vi "Update Named Tag.vi"(7 "Index":i32, 8 "error in (no error)":errorcluster, 9 "Variant":variant, 10 "Tag Name":string, 11 "Raw Message in":refnum<class "Raw Message.lvclass">) -> (0 "error out":errorcluster, 2 "Key not found?":bool, 3 "Raw Message out":refnum<class "Raw Message.lvclass">)   [LabVIEW 2020]
uses:
  Raw Message.lvclass/Raw Message.ctl
  Tag/Basic Type.lvclass
  Raw Message.lvclass
  E:/Labview/LV 2020/Libs/LV Protobuf Raw/Source/Tag/Basic Type.lvclass
  E:/Labview/LV 2020/Libs/LV Protobuf Raw/Source/Proto Value/Proto Type.lvclass
  E:/Labview/LV 2020/Libs/LV Protobuf Raw/Source/Type Serializer/Type Serializer.lvclass
  E:/Labview/LV 2020/Libs/LV Protobuf Raw/Source/String Representable/String Representable.lvclass
  E:/Labview/LV 2020/Libs/LV Protobuf Raw/Source/Wire Type Group/Wire Type Group.lvclass
  E:/Labview/LV 2020/Libs/LV Protobuf Raw/Source/LEN Encoder/LEN.lvclass
  E:/Labview/LV 2020/Libs/LV Protobuf Raw/Source/Message/Raw Message.lvclass
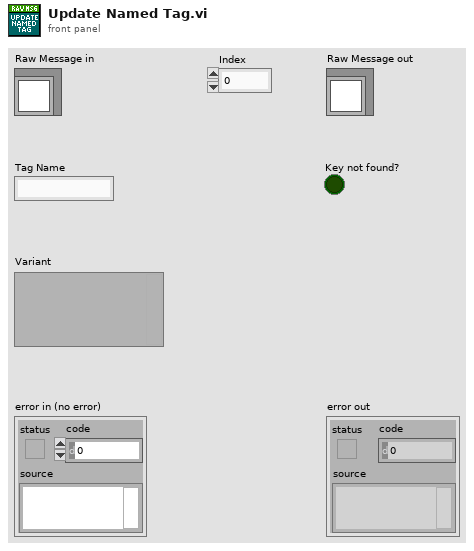
[diagram p1: front panel]
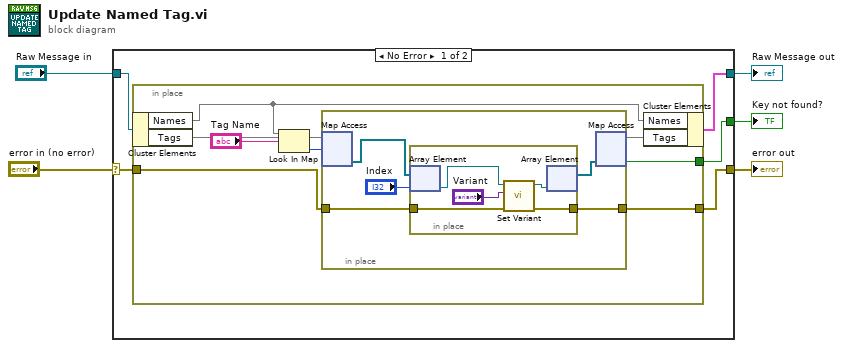
[diagram p0: block diagram]
diagram:
  n1 = case shown="No Error" "error in (no error)" {
    selector: "error in (no error)" -> [w8 w30]
    tunnel: [w7 w30] -> w4
    tunnel: [w9 w29] -> w2
    tunnel: "Raw Message in" -> [w10 w29]
    tunnel: [w6 _] -> w1
    frame No Error {
      n2 = in-place {
        in-place-border: w8 -> [w16]
        in-place-border: [w15] -> w7
        in-place-border: [w14] -> w6
        n3 = in-place-cluster #1(w10) -> ("Names"=w13, "Tags"=w18)
        n4 = Look In Map(map=w13, key="Tag Name") -> (value=w11:u32)  [unwired: 1 in, 1 out]
        n5 = in-place {
          in-place-border: w16 -> [w21]
          in-place-border: [w20] -> w15
          n6 = in-place-map #2(w18, w11) -> (w23:refnum<class "Basic Type.lvclass">[])  [unwired: 1 in, 1 out]
          n7 = in-place {
            in-place-border: w21 -> [w25]
            in-place-border: [w24] -> w20
            n8 = in-place-array #3(w23, "Index") -> (w28:refnum<class "Basic Type.lvclass">)
            n9 = call-dynamic "Set Variant.vi"("error in (no error)"=w25, "Variant"="Variant", "Type Serializer in"=w28) -> ("error out"=w24:errorcluster, "Type Serializer out"=w27:refnum<class "Basic Type.lvclass">)  [unwired: 7 in]
            n10 = in-place-array #3(w27) -> (w22:refnum<class "Basic Type.lvclass">[])  [unwired: 1 out]
          }
          n11 = in-place-map #2(w22) -> (w17:map{u32, refnum<class "Basic Type.lvclass">[]}, w14:bool)  [unwired: 1 in, 1 out]
        }
        n12 = in-place-cluster #1("Names"=w13, "Tags"=w17) -> (w9:cluster{})
      }
    }
    frame Error {
    }
  }
  "error out" <- w4
  "Raw Message out" <- w2
  "Key not found?" <- w1
